vi "自我介绍.vi"(8 "error in (no error)":errorcluster caption="错误输入（无错误）", 11 "橡皮鸭 输入":refnum<class "橡皮鸭.lvclass">) -> (0 "error out":errorcluster caption="错误输出", 3 "橡皮鸭 输出":refnum<class "橡皮鸭.lvclass">)   [LabVIEW 2022 SP3, in "鸭子库.lvlib" / "橡皮鸭.lvclass"]
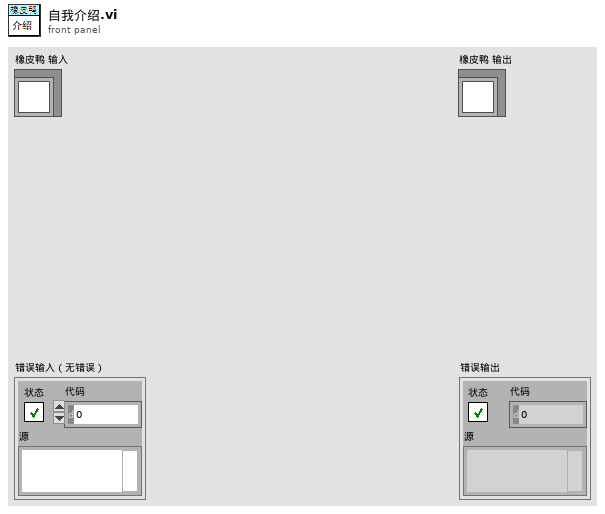
[diagram p1: front panel]
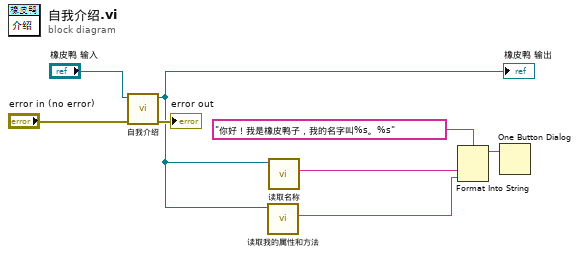
[diagram p0: block diagram]
diagram:
  n1 = call-parent "自我介绍.vi"("error in (no error)"="error in (no error)", "鸭子 输入"="橡皮鸭 输入") -> ("error out"=→"error out":errorcluster, "鸭子 输出"=w2:refnum<class "橡皮鸭.lvclass">)  [unwired: 8 in]
  "橡皮鸭 输出" <- w2
  n2 = call "读取我的属性和方法.vi"("鸭子输入"=w2) -> ("我的属性和方法"=w3:string)  [unwired: 8 in, 2 out]
  n3 = call "读取名称.vi"("鸭子库.lvlib:鸭子.lvclass"=w2) -> ("名称"=w1:string)  [unwired: 8 in, 2 out]
  n4 = Format Into String(format string="你好！我是橡皮鸭子，我的名字叫%s。%s" ("格式字符串"), w1, w3) -> (resulting string=w4:string)  [unwired: 2 in, 1 out]
  n5 = One Button Dialog(message=w4) -> ()  [unwired: 1 in, 1 out]
